vi "Add to DataBase.vi"(8 "error in (no error)":errorcluster, 11 "Object DAO JSON in":refnum<class "Object DAO JSON.lvclass">) -> (0 "error out":errorcluster, 3 "Object DAO JSON out":refnum<class "Object DAO JSON.lvclass">)   [LabVIEW 2020, in "Object DAO JSON.lvclass"]
uses:
  Object DAO JSON.lvclass
  Object DAO JSON.lvclass/Object DAO JSON.ctl
  <vilib>/JDP Science/JSONtext/String Subset.vi
  <vilib>/JDP Science/JSONtext/Parsing/Parse Full Path or Item Name.vi
  <vilib>/JDP Science/JSONtext/Next JSON Value.vi
  <vilib>/JDP Science/JSONtext/support/Error Cluster From Code.vi
  <vilib>/JDP Science/JSONtext/Offset/Find Item Locations by Path.vi
  <vilib>/JDP Science/JSONtext/JSONtext.lvlib
  External Libraries/JSON File Manipulation.lvlibp
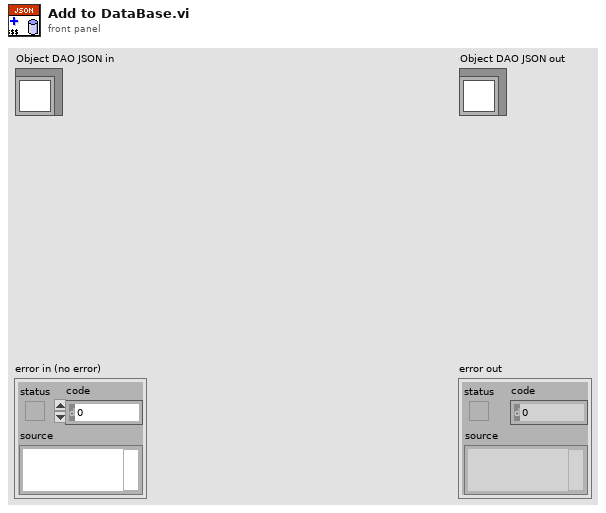
[diagram p1: front panel]
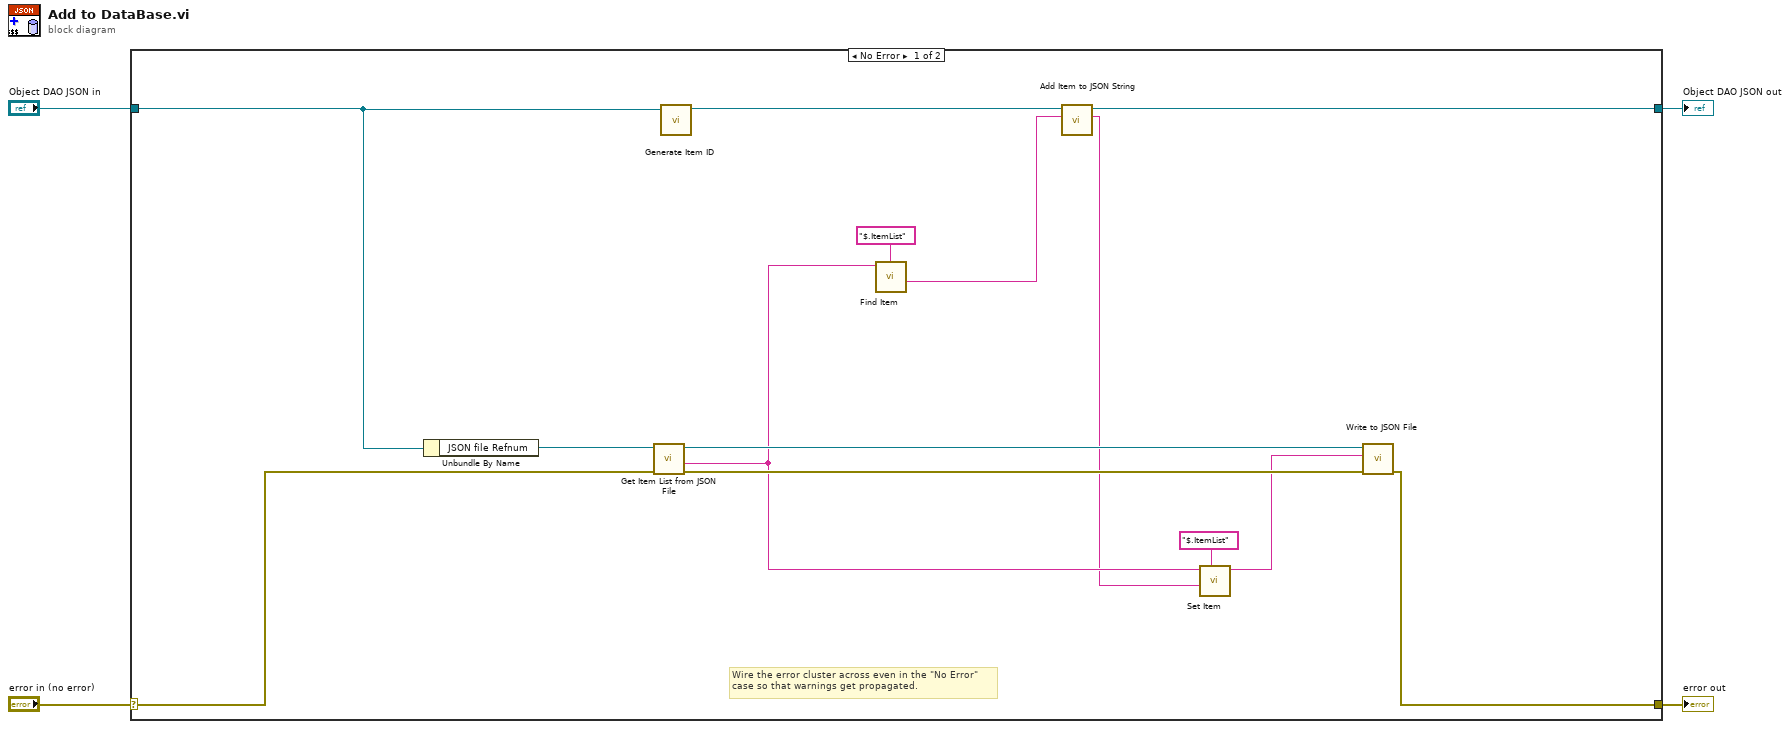
[diagram p0: block diagram]
diagram:
  n1 = case shown="No Error" "error in (no error)" {
    selector: "error in (no error)" -> [w7 w20]
    tunnel: [w6 w20] -> w3
    tunnel: [w5 w19] -> w1
    tunnel: "Object DAO JSON in" -> [w8 w19]
    frame No Error {
      # "Wire the error cluster across even in the \"No Error\"\ncase so that warnings get propagated."
      n2 = Unbundle By Name(w8) -> ("JSON file Refnum"=w18:refnum<file>)
      n3 = call "Get Item List from JSON File.vi"("error in (no error)"=w7, "Byte Stream File in"=w18) -> ("error out"=w17:errorcluster, "JSON String"=w15:string, "Byte Stream File out"=w16:refnum<file>)  [unwired: 6 in, 1 out]
      n4 = call "Generate Item ID.vi"("Customer DAO In"=w8) -> ("Customer DAO Out"=w9:refnum<class "Object DAO JSON.lvclass">)  [unwired: 10 in]
      n5 = call <vilib>:"Find Item.vi"("$Path or Item Name"="$.ItemList", "JSON"=w15) -> ("<JSON>"=w11:string)  [unwired: 6 in, 3 out]
      n6 = call "Add Item to JSON String.vi"("JSON String In"=w11, "Customer DAO JSON in"=w9) -> ("JSON string out"=w10:string, "Customer DAO JSON out"=w5:refnum<class "Object DAO JSON.lvclass">)  [unwired: 8 in]
      n7 = call <vilib>:"Set Item.vi"("$Path or Item Name"="$.ItemList", "JSON to Insert"=w10, "JSON"=w15) -> ("<JSON>"=w13:string)  [unwired: 5 in, 2 out]
      n8 = call "Write to JSON File.vi"("error in (no error)"=w17, "JSON String"=w13, "Byte Stream File in"=w16) -> ("error out"=w6:errorcluster)  [unwired: 8 in]
    }
    frame Error {
    }
  }
  "error out" <- w3
  "Object DAO JSON out" <- w1
